vi "Configure Channels (5752).vi"(8 "error in":errorcluster, 10 "Channel Selector":T1={"First Channel"=enum."Channel 0", "Second Channel"=enum."Channel 1"}, 11 "FPGA VI Reference In":refnum<k20>) -> (0 "error out":errorcluster, 3 "FPGA VI Reference Out":refnum<k20>)   [LabVIEW 2012]
uses:
  <vilib>/Utility/error.llb/Error Cluster From Error Code.vi
  <vilib>/rvi/errors/niLvFpgaAdjustHostInterfaceError.vi
  <vilib>/rvi/interface/nirviReadWriteControl/nirviReadWriteControl.xnode
  NiFpgaLv.dll
  <vilib>/rvi/interface/Simulation/niFpgaSimulationCallBeginRW.vi
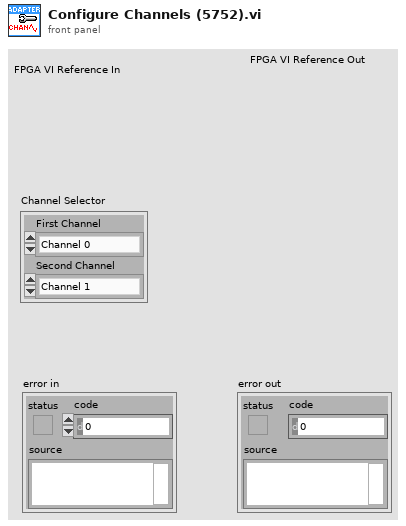
[diagram p1: front panel]
types:
  T1 = cluster{"First Channel":enum16{"Channel 0", "Channel 1", "Channel 2", "Channel 3"}, "Second Channel":enum16{"Channel 0", "Channel 1", "Channel 2", "Channel 3"}}
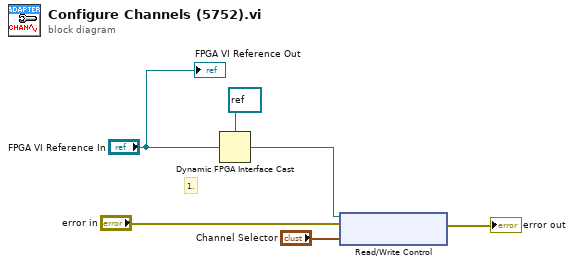
[diagram p0: block diagram]
diagram:
  # "1."
  n1 = Dynamic FPGA Interface Cast(Session In=refnum<k20> refnum ("Type"), Type="FPGA VI Reference In") -> (Session Out=w4:refnum<k20>)
  n2 = xnode "Read/Write Control"("FPGA VI Reference In"=w4, "error in"="error in", "Channel Selector"="Channel Selector") -> ("error out"=→"error out":errorcluster)  [unwired: 1 out]
  "FPGA VI Reference Out" <- "FPGA VI Reference In"
